vi "Monitoring task.vi"   [LabVIEW 2016]
types:
  T1 = enum16{"启动测量", "标样核查", "零点核查", "跨度核查", "空白测试", "平行样测试", "加标回收", "空白校准", "标样校准", "初始化（清洗）", "停止测试", "仪器重启", "校时", "模式设置", "测量间隔设置"}
  T2 = cluster{"测试模式":enum16{"水样测试", "平行样测试", "集成干预测试", "加标回收"}, "参数启用":cluster{"氨氮":bool, "总磷":bool, "总氮":bool, "多参数":bool, "CODMn":bool, "CODcr":bool, "超标留样":bool}}
  T3 = cluster{"启动参数":cluster{"氨氮":bool, "总磷":bool, "总氮":bool, "CODMn":bool, "CODCr":bool, "多参数":bool}, "运行模式":enum16{"维护模式", "常规模式", "应急模式", "质控模式"}, "质控频次":enum16{"关闭", "每天", "星期一", "星期二", "星期三", "星期四", "星期五", "星期六", "星期日"}, "空白核查时间":u16, "跨度核查时间":u16, "多参数测试间隔":u16, "湿化学测试间隔":u16}
  T4 = typedef "质控单元V4.lvlib/测试子流程.ctl" = enum16{"水样测试（润洗采样分开）", "水样测试（润洗采样合并）", "水样测试（不启动采配水）", "加标回收（润洗采样分开）", "加标回收（润洗采样合并）", "加标回收（不启动采配水）", "集成干预测试", "平行样测试", "平行样测试（不启动采配水）", "水样测试（不含采样杯）", "平行样测试（不含采样杯）", "集成干预测试（不含采样杯）"}
  T5 = typedef "质控单元V4.lvlib/质控slave id.ctl" = enum16{"null", "氨氮", "总磷", "总氮", "CODMn", "CODCr", "氟化物"}
  T6 = cluster{"氨氮":enum16{"直接采样", "采样杯采样"}, "总磷":enum16{"直接采样", "采样杯采样"}, "总氮":enum16{"直接采样", "采样杯采样"}, "CODMn":enum16{"直接采样", "采样杯采样"}, "CODCr":enum16{"直接采样", "采样杯采样"}}
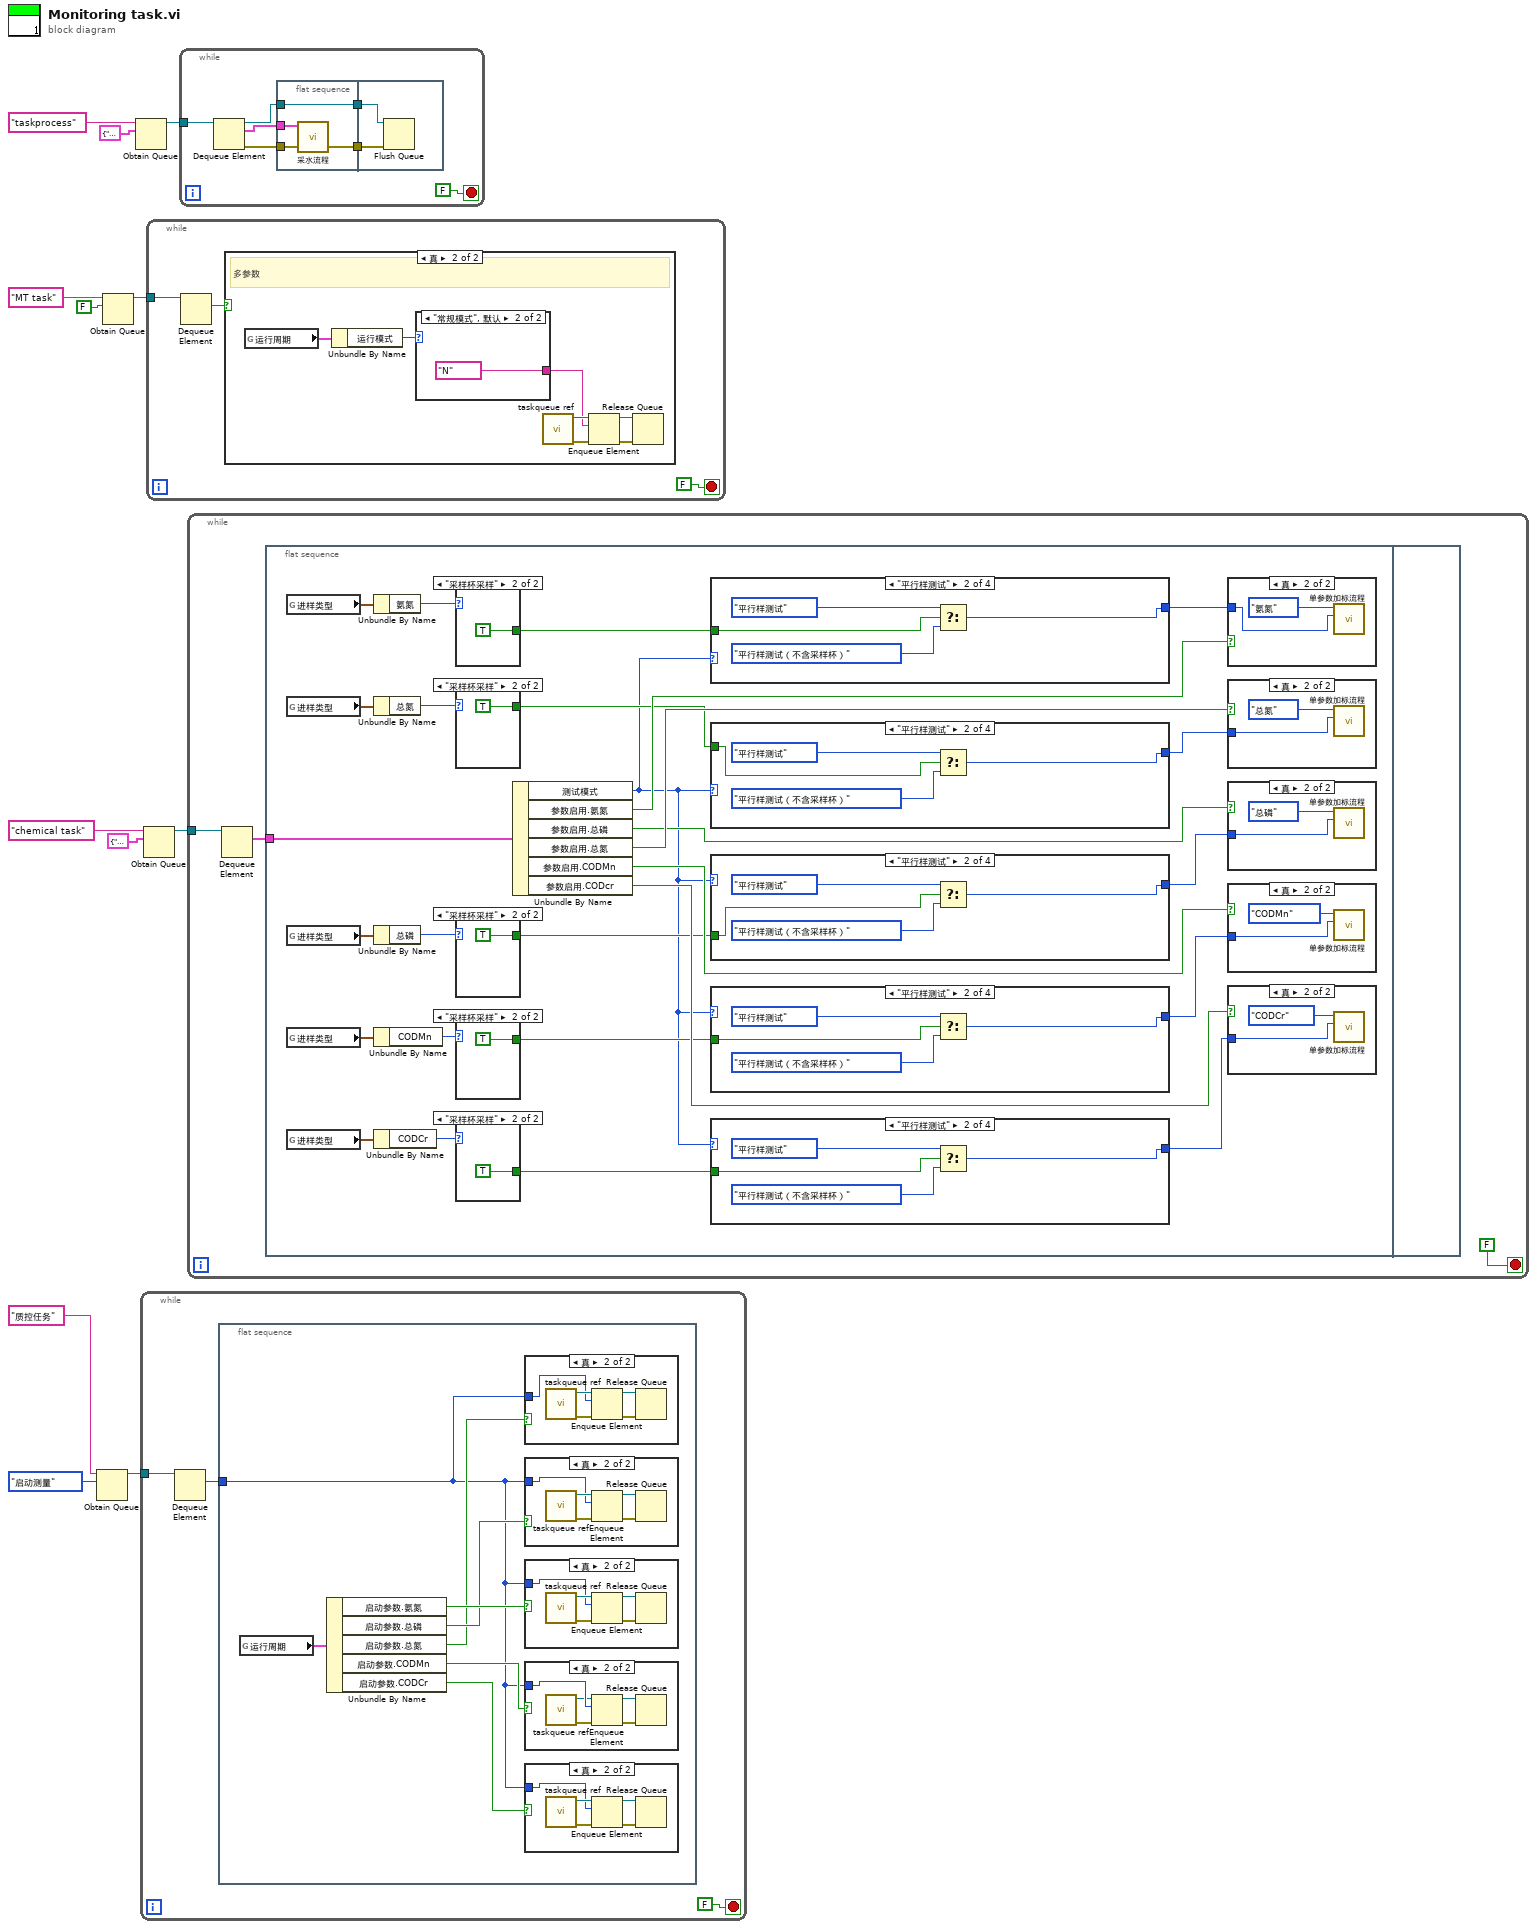
[diagram p0: block diagram]
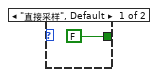
[diagram p7: hidden frame]
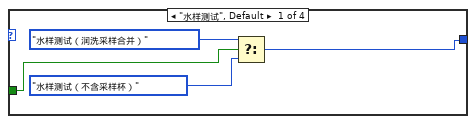
[diagram p8: hidden frame]
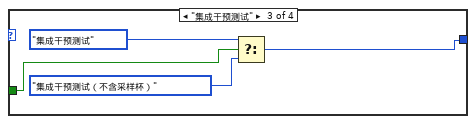
[diagram p9: hidden frame]
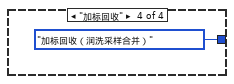
[diagram p10: hidden frame]
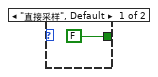
[diagram p11: hidden frame]
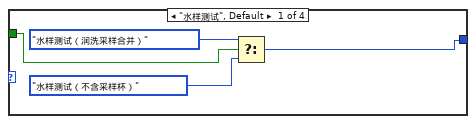
[diagram p12: hidden frame]
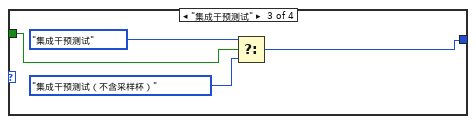
[diagram p13: hidden frame]
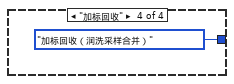
[diagram p14: hidden frame]
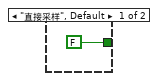
[diagram p15: hidden frame]
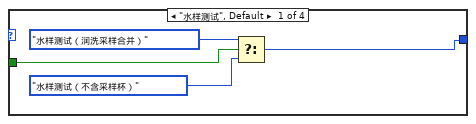
[diagram p16: hidden frame]
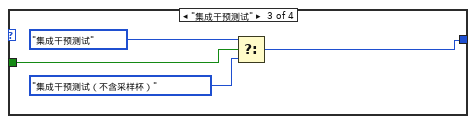
[diagram p17: hidden frame]
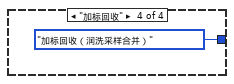
[diagram p18: hidden frame]
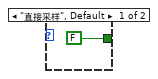
[diagram p19: hidden frame]
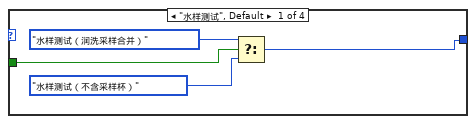
[diagram p20: hidden frame]
diagram:
  n1 = Obtain Queue(name (unnamed)="质控任务" ("名称（未命名）"), element data type=T1."启动测量" ("控制命令")) -> (queue out=w1:refnum<queue>)  [unwired: 3 in, 2 out]
  n2 = Obtain Queue(name (unnamed)="MT task" ("名称（未命名）"), element data type=FALSE) -> (queue out=w9:refnum<queue>)  [unwired: 3 in, 2 out]
  n3 = Obtain Queue(name (unnamed)="taskprocess" ("名称（未命名）"), element data type=T2 {"测试模式"=enum."水样测试", "参数启用"={"氨氮"=FALSE, "总磷"=FALSE, "总氮"=FALSE, "多参数"=FALSE, "CODMn"=FALSE, "CODcr"=FALSE, "超标留样"=FALSE}} ("参数")) -> (queue out=w6:refnum<queue>)  [unwired: 3 in, 2 out]
  n4 = while {
    tunnel: w1 -> [w14]
    stop <- FALSE stop-if-true
    n5 = Dequeue Element(queue=w14) -> (element=w13:T1)  [unwired: 2 in, 3 out]
    n6 = flat-sequence {
      tunnel: w13 -> [w16]
      frame #0 {
        n7 = global read "系统设置全局变量.vi" "运行周期"() -> (w22:T3)
        n8 = Unbundle By Name(w22) -> ("启动参数.氨氮"=w21:bool, "启动参数.总磷"=w20:bool, "启动参数.总氮"=w19:bool, "启动参数.CODMn"=w18:bool, "启动参数.CODCr"=w17:bool)
        n9 = case shown="真" w19 {
          tunnel: w16 -> [_ w33]
          frame False {
          }
          frame True {
            n10 = call "taskqueue ref.vi"() -> ("错误输出"=w35:errorcluster, "队列输出"=w34:refnum<queue>)  [unwired: 10 in]
            n11 = Enqueue Element(queue=w34, element=w33, error in (no error)=w35) -> (queue out=w36:refnum<queue>, error out=w37:errorcluster)  [unwired: 1 in, 1 out]
            n12 = Release Queue(queue=w36, error in (no error)=w37) -> ()  [unwired: 1 in, 3 out]
          }
        }
        n13 = case shown="真" w20 {
          tunnel: w16 -> [_ w38]
          frame False {
          }
          frame True {
            n14 = call "taskqueue ref.vi"() -> ("错误输出"=w39:errorcluster, "队列输出"=w40:refnum<queue>)  [unwired: 10 in]
            n15 = Enqueue Element(queue=w40, element=w38, error in (no error)=w39) -> (queue out=w42:refnum<queue>, error out=w41:errorcluster)  [unwired: 1 in, 1 out]
            n16 = Release Queue(queue=w42, error in (no error)=w41) -> ()  [unwired: 1 in, 3 out]
          }
        }
        n17 = case shown="真" w21 {
          tunnel: w16 -> [_ w43]
          frame False {
          }
          frame True {
            n18 = call "taskqueue ref.vi"() -> ("错误输出"=w44:errorcluster, "队列输出"=w45:refnum<queue>)  [unwired: 10 in]
            n19 = Enqueue Element(queue=w45, element=w43, error in (no error)=w44) -> (queue out=w47:refnum<queue>, error out=w46:errorcluster)  [unwired: 1 in, 1 out]
            n20 = Release Queue(queue=w47, error in (no error)=w46) -> ()  [unwired: 1 in, 3 out]
          }
        }
        n21 = case shown="真" w18 {
          tunnel: w16 -> [_ w30]
          frame False {
          }
          frame True {
            n22 = call "taskqueue ref.vi"() -> ("错误输出"=w28:errorcluster, "队列输出"=w29:refnum<queue>)  [unwired: 10 in]
            n23 = Enqueue Element(queue=w29, element=w30, error in (no error)=w28) -> (queue out=w31:refnum<queue>, error out=w32:errorcluster)  [unwired: 1 in, 1 out]
            n24 = Release Queue(queue=w31, error in (no error)=w32) -> ()  [unwired: 1 in, 3 out]
          }
        }
        n25 = case shown="真" w17 {
          tunnel: w16 -> [_ w23]
          frame False {
          }
          frame True {
            n26 = call "taskqueue ref.vi"() -> ("错误输出"=w24:errorcluster, "队列输出"=w25:refnum<queue>)  [unwired: 10 in]
            n27 = Enqueue Element(queue=w25, element=w23, error in (no error)=w24) -> (queue out=w27:refnum<queue>, error out=w26:errorcluster)  [unwired: 1 in, 1 out]
            n28 = Release Queue(queue=w27, error in (no error)=w26) -> ()  [unwired: 1 in, 3 out]
          }
        }
      }
    }
  }
  n29 = Obtain Queue(name (unnamed)="chemical task" ("名称（未命名）"), element data type=T2 {"测试模式"=enum."水样测试", "参数启用"={"氨氮"=FALSE, "总磷"=FALSE, "总氮"=FALSE, "多参数"=FALSE, "CODMn"=FALSE, "CODcr"=FALSE, "超标留样"=FALSE}} ("参数")) -> (queue out=w11:refnum<queue>)  [unwired: 3 in, 2 out]
  n30 = while {
    tunnel: w9 -> [w50]
    stop <- FALSE stop-if-true
    n31 = Dequeue Element(queue=w50) -> (element=w49:bool)  [unwired: 2 in, 3 out]
    n32 = case shown="真" w49 {
      frame False {
        (unwired) TRUE ("t")
      }
      frame True {
        # "多参数"
        n33 = global read "系统设置全局变量.vi" "运行周期"() -> (w57:T3)
        n34 = Unbundle By Name(w57) -> ("运行模式"=w56:enum16{"维护模式", "常规模式", "应急模式", "质控模式"})
        n35 = case shown="\"常规模式\", 默认" w56 {
          tunnel: ["M" ("数据标记表") "N" ("数据标记表")] -> w51
          frame "维护模式" {
          }
          frame "常规模式", Default {
          }
        }
        n36 = call "taskqueue ref.vi"() -> ("错误输出"=w53:errorcluster, "队列输出"=w52:refnum<queue>)  [unwired: 10 in]
        n37 = Enqueue Element(queue=w52, element=w51, error in (no error)=w53) -> (queue out=w54:refnum<queue>, error out=w55:errorcluster)  [unwired: 1 in, 1 out]
        n38 = Release Queue(queue=w54, error in (no error)=w55) -> ()  [unwired: 1 in, 3 out]
      }
    }
  }
  n39 = while {
    tunnel: w6 -> [w66]
    stop <- FALSE stop-if-true
    n40 = Dequeue Element(queue=w66) -> (queue out=w63:refnum<queue>, element=w64:T2, error out=w60:errorcluster)  [unwired: 2 in, 1 out]
    n41 = flat-sequence {
      tunnel: w64 -> [w69]
      tunnel: w63 -> [w68]
      tunnel: [w68] -> w62
      tunnel: [w67] -> w61
      tunnel: w60 -> [w67]
      tunnel: w62 -> [w71]
      tunnel: w61 -> [w70]
      frame #0 {
        n42 = call "采水流程.vi"("参数"=w69) -> ()  [unwired: 11 in]
      }
      frame #1 {
        n43 = Flush Queue(queue=w71, error in (no error)=w70) -> ()  [unwired: 3 out]
      }
    }
  }
  n44 = while {
    tunnel: w11 -> [w74]
    stop <- FALSE stop-if-true
    n45 = Dequeue Element(queue=w74) -> (element=w73:T2)  [unwired: 2 in, 3 out]
    n46 = flat-sequence {
      tunnel: w73 -> [w101]
      frame #0 {
        n47 = global read "系统设置全局变量.vi" "进样类型"() -> (w93:T6)
        n48 = global read "系统设置全局变量.vi" "进样类型"() -> (w83:T6)
        n49 = global read "系统设置全局变量.vi" "进样类型"() -> (w80:T6)
        n50 = global read "系统设置全局变量.vi" "进样类型"() -> (w90:T6)
        n51 = global read "系统设置全局变量.vi" "进样类型"() -> (w86:T6)
        n52 = Unbundle By Name(w93) -> ("氨氮"=w92:enum16{"直接采样", "采样杯采样"})
        n53 = Unbundle By Name(w83) -> ("总氮"=w84:enum16{"直接采样", "采样杯采样"})
        n54 = Unbundle By Name(w80) -> ("总磷"=w79:enum16{"直接采样", "采样杯采样"})
        n55 = Unbundle By Name(w90) -> ("CODMn"=w91:enum16{"直接采样", "采样杯采样"})
        n56 = Unbundle By Name(w86) -> ("CODCr"=w85:enum16{"直接采样", "采样杯采样"})
        n57 = case shown="\"采样杯采样\"" w92 {
          tunnel: [FALSE TRUE] -> w94
          frame "直接采样", Default {
          }
          frame "采样杯采样" {
          }
        }
        n58 = case shown="\"采样杯采样\"" w84 {
          tunnel: [FALSE TRUE] -> w82
          frame "直接采样", Default {
          }
          frame "采样杯采样" {
          }
        }
        n59 = case shown="\"采样杯采样\"" w79 {
          tunnel: [FALSE TRUE] -> w81
          frame "直接采样", Default {
          }
          frame "采样杯采样" {
          }
        }
        n60 = case shown="\"采样杯采样\"" w91 {
          tunnel: [FALSE TRUE] -> w89
          frame "直接采样", Default {
          }
          frame "采样杯采样" {
          }
        }
        n61 = case shown="\"采样杯采样\"" w85 {
          tunnel: [FALSE TRUE] -> w87
          frame "直接采样", Default {
          }
          frame "采样杯采样" {
          }
        }
        n62 = Unbundle By Name(w101) -> ("测试模式"=w75:enum16{"水样测试", "平行样测试", "集成干预测试", "加标回收"}, "参数启用.氨氮"=w100:bool, "参数启用.总磷"=w96:bool, "参数启用.总氮"=w99:bool, "参数启用.CODMn"=w98:bool, "参数启用.CODcr"=w97:bool)
        n63 = case shown="\"平行样测试\"" w75 {
          tunnel: w94 -> [w167 w171 w175 _]
          tunnel: [w164 w168 w172 测试子流程."加标回收（润洗采样合并）" ("流程类型")] -> w95
          frame "水样测试", Default {
            n64 = Select(t=测试子流程."水样测试（润洗采样合并）" ("流程类型"), s=w167, f=测试子流程."水样测试（不含采样杯）" ("流程类型")) -> (s? t:f=w164:T4)
          }
          frame "平行样测试" {
            n65 = Select(t=测试子流程."平行样测试" ("流程类型"), s=w171, f=测试子流程."平行样测试（不含采样杯）" ("流程类型")) -> (s? t:f=w168:T4)
          }
          frame "集成干预测试" {
            n66 = Select(t=测试子流程."集成干预测试" ("流程类型"), s=w175, f=测试子流程."集成干预测试（不含采样杯）" ("流程类型")) -> (s? t:f=w172:T4)
          }
          frame "加标回收" {
          }
        }
        n67 = case shown="\"平行样测试\"" w75 {
          tunnel: w82 -> [w122 w126 w130 _]
          tunnel: [w119 w123 w127 测试子流程."加标回收（润洗采样合并）" ("流程类型")] -> w77
          frame "水样测试", Default {
            n68 = Select(t=测试子流程."水样测试（润洗采样合并）" ("流程类型"), s=w122, f=测试子流程."水样测试（不含采样杯）" ("流程类型")) -> (s? t:f=w119:T4)
          }
          frame "平行样测试" {
            n69 = Select(t=测试子流程."平行样测试" ("流程类型"), s=w126, f=测试子流程."平行样测试（不含采样杯）" ("流程类型")) -> (s? t:f=w123:T4)
          }
          frame "集成干预测试" {
            n70 = Select(t=测试子流程."集成干预测试" ("流程类型"), s=w130, f=测试子流程."集成干预测试（不含采样杯）" ("流程类型")) -> (s? t:f=w127:T4)
          }
          frame "加标回收" {
          }
        }
        n71 = case shown="\"平行样测试\"" w75 {
          tunnel: w81 -> [w107 w111 w115 _]
          tunnel: [w104 w108 w112 测试子流程."加标回收（润洗采样合并）" ("流程类型")] -> w76
          frame "水样测试", Default {
            n72 = Select(t=测试子流程."水样测试（润洗采样合并）" ("流程类型"), s=w107, f=测试子流程."水样测试（不含采样杯）" ("流程类型")) -> (s? t:f=w104:T4)
          }
          frame "平行样测试" {
            n73 = Select(t=测试子流程."平行样测试" ("流程类型"), s=w111, f=测试子流程."平行样测试（不含采样杯）" ("流程类型")) -> (s? t:f=w108:T4)
          }
          frame "集成干预测试" {
            n74 = Select(t=测试子流程."集成干预测试" ("流程类型"), s=w115, f=测试子流程."集成干预测试（不含采样杯）" ("流程类型")) -> (s? t:f=w112:T4)
          }
          frame "加标回收" {
          }
        }
        n75 = case shown="\"平行样测试\"" w75 {
          tunnel: w89 -> [w152 w156 w160 _]
          tunnel: [w149 w153 w157 测试子流程."加标回收（润洗采样合并）" ("流程类型")] -> w88
          frame "水样测试", Default {
            n76 = Select(t=测试子流程."水样测试（润洗采样合并）" ("流程类型"), s=w152, f=测试子流程."水样测试（不含采样杯）" ("流程类型")) -> (s? t:f=w149:T4)
          }
          frame "平行样测试" {
            n77 = Select(t=测试子流程."平行样测试" ("流程类型"), s=w156, f=测试子流程."平行样测试（不含采样杯）" ("流程类型")) -> (s? t:f=w153:T4)
          }
          frame "集成干预测试" {
            n78 = Select(t=测试子流程."集成干预测试" ("流程类型"), s=w160, f=测试子流程."集成干预测试（不含采样杯）" ("流程类型")) -> (s? t:f=w157:T4)
          }
          frame "加标回收" {
          }
        }
        n79 = case shown="\"平行样测试\"" w75 {
          tunnel: w87 -> [w137 w141 w145 _]
          tunnel: [w134 w138 w142 测试子流程."加标回收（润洗采样合并）" ("流程类型")] -> w78
          frame "水样测试", Default {
            n80 = Select(t=测试子流程."水样测试（润洗采样合并）" ("流程类型"), s=w137, f=测试子流程."水样测试（不含采样杯）" ("流程类型")) -> (s? t:f=w134:T4)
          }
          frame "平行样测试" {
            n81 = Select(t=测试子流程."平行样测试" ("流程类型"), s=w141, f=测试子流程."平行样测试（不含采样杯）" ("流程类型")) -> (s? t:f=w138:T4)
          }
          frame "集成干预测试" {
            n82 = Select(t=测试子流程."集成干预测试" ("流程类型"), s=w145, f=测试子流程."集成干预测试（不含采样杯）" ("流程类型")) -> (s? t:f=w142:T4)
          }
          frame "加标回收" {
          }
        }
        n83 = case shown="真" w100 {
          tunnel: w95 -> [_ w186]
          frame False {
          }
          frame True {
            n84 = call "单参数加标流程.vi"("流程类型"=w186, "Slave ID"=质控slave_id."氨氮") -> ()  [unwired: 10 in]
          }
        }
        n85 = case shown="真" w99 {
          tunnel: w77 -> [_ w182]
          frame False {
          }
          frame True {
            n86 = call "单参数加标流程.vi"("流程类型"=w182, "Slave ID"=质控slave_id."总氮") -> ()  [unwired: 10 in]
          }
        }
        n87 = case shown="真" w96 {
          tunnel: w76 -> [_ w184]
          frame False {
          }
          frame True {
            n88 = call "单参数加标流程.vi"("流程类型"=w184, "Slave ID"=质控slave_id."总磷") -> ()  [unwired: 10 in]
          }
        }
        n89 = case shown="真" w98 {
          tunnel: w88 -> [_ w180]
          frame False {
          }
          frame True {
            n90 = call "单参数加标流程.vi"("流程类型"=w180, "Slave ID"=质控slave_id."CODMn") -> ()  [unwired: 10 in]
          }
        }
        n91 = case shown="真" w97 {
          tunnel: w78 -> [_ w178]
          frame False {
          }
          frame True {
            n92 = call "单参数加标流程.vi"("流程类型"=w178, "Slave ID"=质控slave_id."CODCr") -> ()  [unwired: 10 in]
          }
        }
      }
      frame #1 {
      }
    }
  }
